vi "convert_time_to_voltage.vi"(8 "calibration file":path, 10 "Voltage Divide Factor":dbl, 11 "measurement":dbl) -> (3 "Voltage":dbl)   [LabVIEW 2015]
doc: "Converts a pulse width time to a voltage using calibration measurements stored in CSV files."
uses:
  <vilib>/Utility/file.llb/Read From Spreadsheet File (DBL).vi
  <vilib>/gmath/NI_Gmath.lvlib
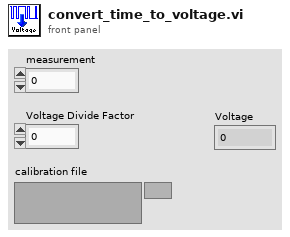
[diagram p1: front panel]
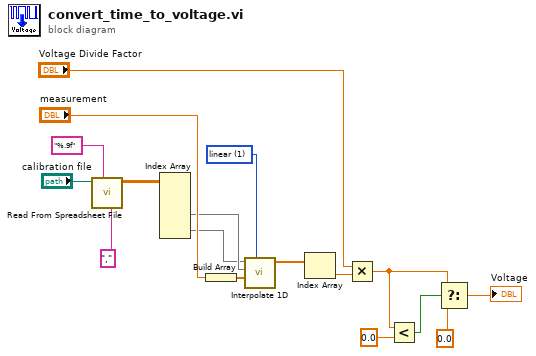
[diagram p0: block diagram]
diagram:
  w17 = 1 items=["nearest", "linear", "spline", "cubic Hermite", "Lagrange"] ("method")
  n1 = call-poly <vilib>:"Read From Spreadsheet File.vi"("delimiter (\\t)"="," ("delimiter (\\t)"), "format (%.3f)"="%.9f", "file path (dialog if empty)"="calibration file") -> ("all rows"=w11:dbl[][])  [unwired: 4 in, 4 out]
  n2 = Index Array(array=w11) -> (element #2=w7:dbl[], element #3=w6:dbl[])  [unwired: 6 in, 1 out]
  n3 = Build Array("measurement") -> (w16:dbl[])
  n4 = call <vilib>:"Interpolate 1D.vi"("method"=w17, "xi"=w16, "X"=w7, "Y"=w6) -> ("yi"=w14:dbl[])  [unwired: 5 in, 2 out]
  n5 = Index Array(array=w14) -> (element=w13:dbl)  [unwired: 1 in]
  n6 = Multiply(x="Voltage Divide Factor", y=w13) -> (x*y=w2:dbl)
  n7 = Less?(x=w2, y=0.0) -> (x < y?=w3:bool)
  n8 = Select(t=w2, s=w3, f=0.0) -> (s? t:f=→"Voltage":dbl)
